vi "TSCAN DBCAnalysisReceive.vi"(0 "路径输入":path, 1 "Message":string, 2 "SignalName":string, 7 "簇":T1, 11 "错误输入（无错误）":errorcluster) -> (4 "路径输出":path, 8 "SigValue":dbl, 15 "错误输出":errorcluster)   [LabVIEW 2013]
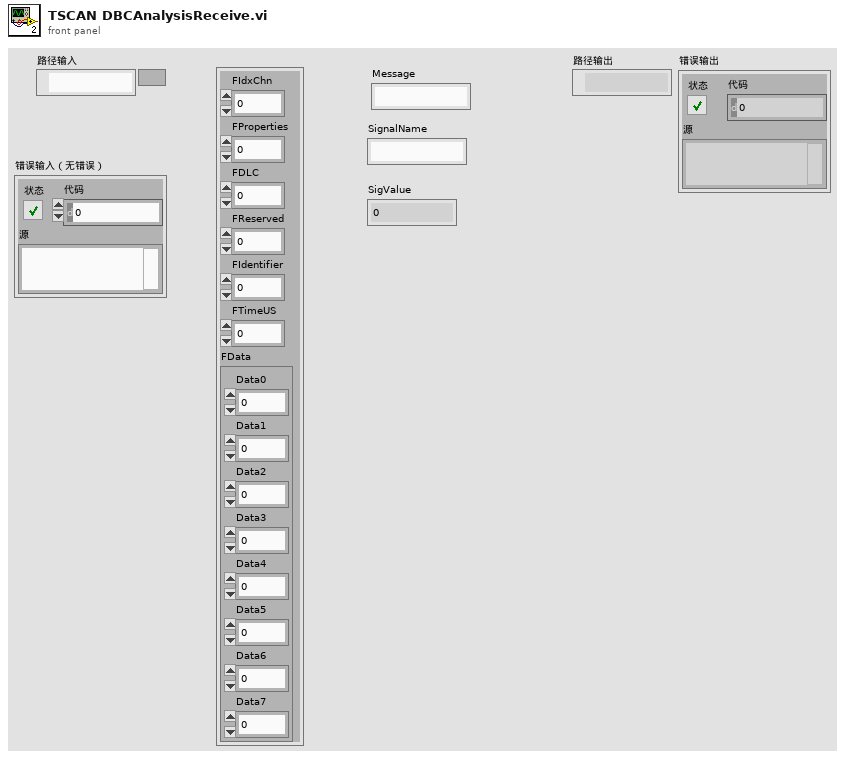
[diagram p1: front panel]
types:
  T1 = cluster{"FIdxChn":u8, "FProperties":u8, "FDLC":u8, "FReserved":u8, "FIdentifier":i32, "FTimeUS":u64, "FData":cluster{"Data0":u8, "Data1":u8, "Data2":u8, "Data3":u8, "Data4":u8, "Data5":u8, "Data6":u8, "Data7":u8}}
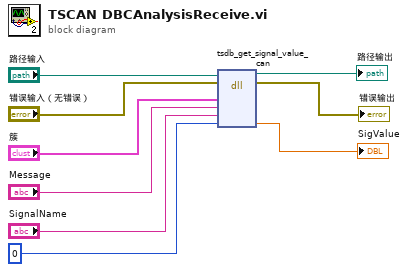
[diagram p0: block diagram]
diagram:
  n1 = dll-call lib="PTH17abs EDemo同星\nTSCAN_V1.0ConfigTSMaster.dll" fn="tsdb_get_signal_value_can"(path in="路径输入", error in="错误输入（无错误）", "CANObJ"="簇", "Message"="Message", "Signal"="SignalName", "SigValue"=0) -> (path out=→"路径输出":path, error out=→"错误输出":errorcluster, "SigValue"=→"SigValue":dbl)  [unwired: 5 in]
